vi "GetRawDataFilePaths.vi"(11 "Results file or Folder":path) -> (3 "RawDataFilePaths":string[](array[string]), 5 "RowNumbers":i32[](array[numeric]))   [LabVIEW 2011]
uses:
  Globals/Constants_global.vi
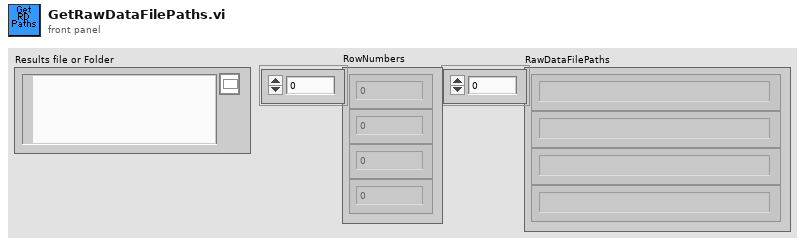
[diagram p1: front panel]
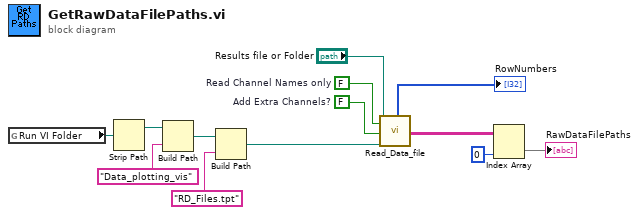
[diagram p0: block diagram]
diagram:
  w9 = FALSE  # Add Extra Channels?
  w8 = FALSE  # Read Channel Names only
  n1 = global read "Constants_global.vi" "Run VI Folder"() -> (w5:path)
  n2 = Strip Path(path=w5) -> (stripped path=w4:path)  [unwired: 1 out]
  n3 = Build Path(base path=w4, name or relative path="Data_plotting_vis") -> (appended path=w3:path)
  n4 = Build Path(base path=w3, name or relative path="RD_Files.tpt") -> (appended path=w7:path)
  n5 = call "Read_Data_file.vi"("Results file"="Results file or Folder", "Read Channel Names only"=w8, "Add Extra Channels?"=w9, "Template File"=w7) -> ("Row numbers"=→"RowNumbers":i32[], "Channel Values Out"=w13:string[][])  [unwired: 1 in, 13 out]
  n6 = Index Array(array=w13, index (col)=0 ("index (row)")) -> (element=→"RawDataFilePaths":string[])  [unwired: 1 in]
